vi "Send Reference.vi"(8 "error in (no error)":errorcluster, 11 "Sync Box in":refnum<class "Sync Box.lvclass">) -> (0 "error out":errorcluster, 3 "Sync Box out":refnum<class "Sync Box.lvclass">)   [LabVIEW 2012, in "Sync Box.lvclass"]
uses:
  Sync Box.lvclass
  Sync Box.lvclass/Sync Box.ctl
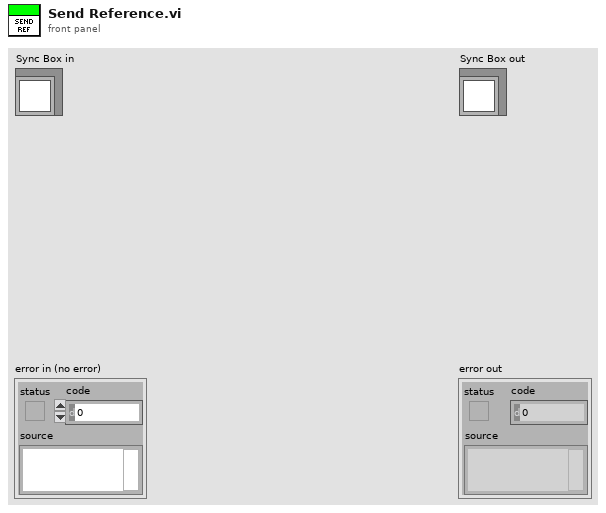
[diagram p1: front panel]
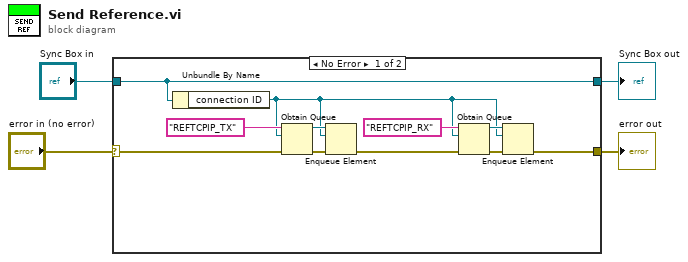
[diagram p0: block diagram]
diagram:
  n1 = case shown="No Error" "error in (no error)" {
    selector: "error in (no error)" -> [w11 w17]
    tunnel: [w6 w17] -> w3
    tunnel: [w15 w16] -> w1
    tunnel: "Sync Box in" -> [w15 w16]
    frame No Error {
      n2 = Unbundle By Name(w15) -> ("connection ID"=w5:refnum<k5>)
      n3 = Obtain Queue(name (unnamed)="REFTCPIP_TX", element data type=w5, error in (no error)=w11) -> (queue out=w13:refnum<queue>, error out=w12:errorcluster)  [unwired: 2 in, 1 out]
      n4 = Enqueue Element(queue=w13, element=w5, error in (no error)=w12) -> (error out=w7:errorcluster)  [unwired: 1 in, 2 out]
      n5 = Obtain Queue(name (unnamed)="REFTCPIP_RX", element data type=w5, error in (no error)=w7) -> (queue out=w9:refnum<queue>, error out=w10:errorcluster)  [unwired: 2 in, 1 out]
      n6 = Enqueue Element(queue=w9, element=w5, error in (no error)=w10) -> (error out=w6:errorcluster)  [unwired: 1 in, 2 out]
    }
    frame Error {
    }
  }
  "error out" <- w3
  "Sync Box out" <- w1
